vi "Report Get Gage Data.vi"(10 "Gage Data":string[][](array[string]), 11 "Array":dbl[][](array[numeric])) -> (1 "Array 2":i32[][](array[numeric]), 2 "Variant":variant, 3 "Array 3":string[][](array[string]))   [LabVIEW 2020]
uses:
  <vilib>/Analysis/baseanly.llb/Mean (DBL).vi
  <vilib>/Analysis/NI_AALBase.lvlib
panel:
  out "Variant 2":variant
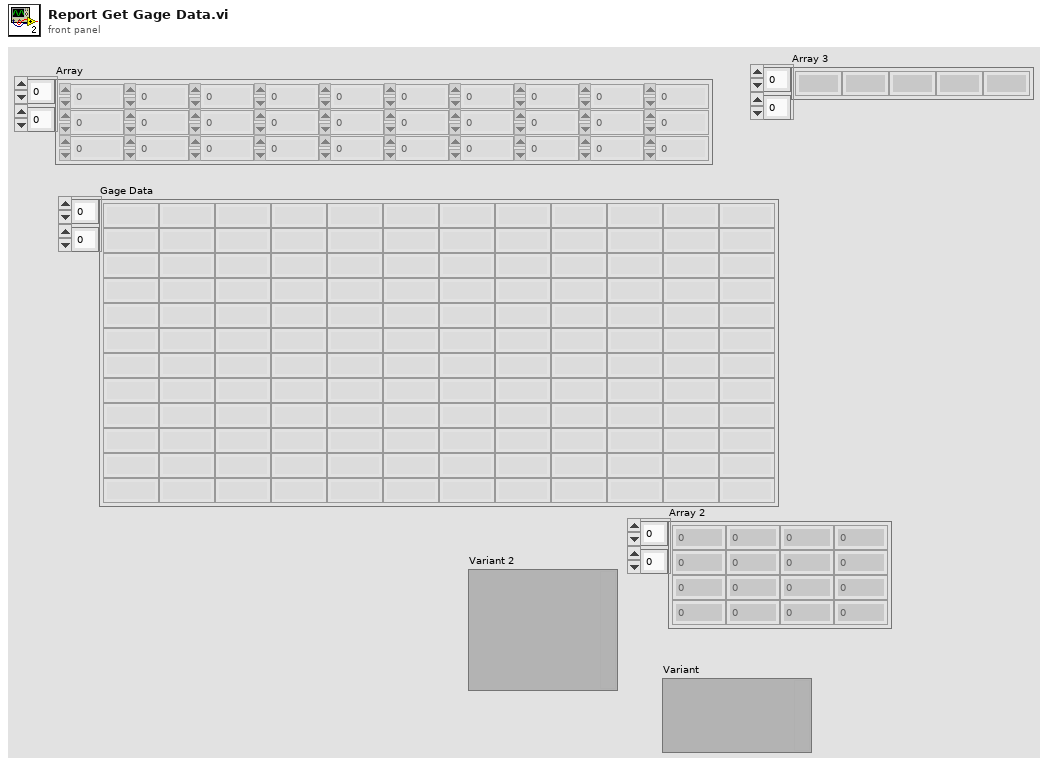
[diagram p1: front panel]
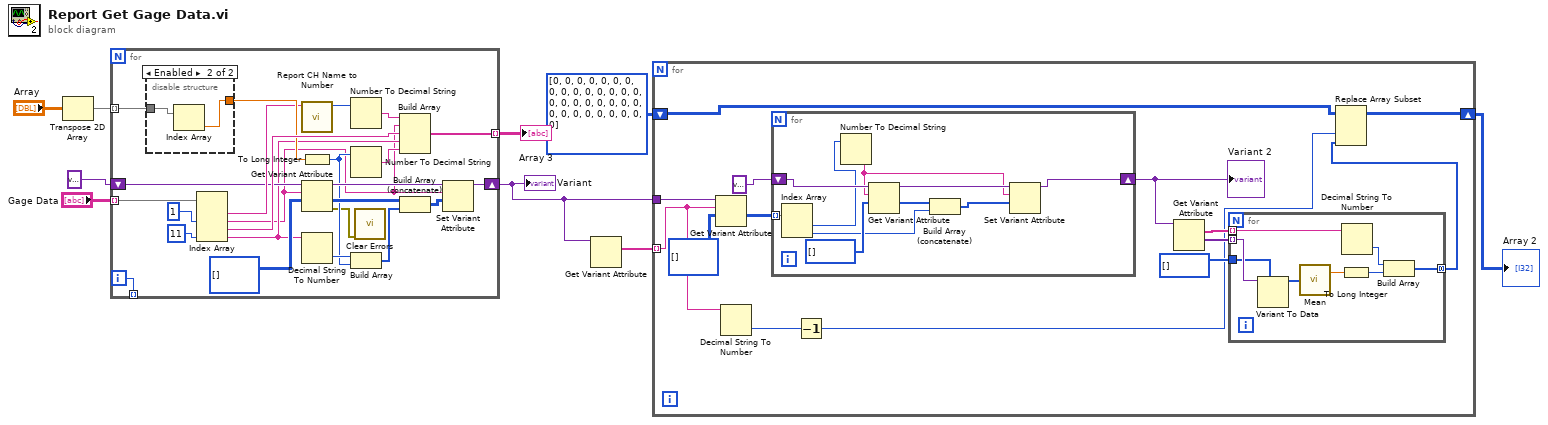
[diagram p0: block diagram]
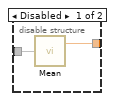
[diagram p2: hidden frame]
diagram:
  n1 = Transpose 2D Array(2D array="Array") -> (transposed array=w7:dbl[][])
  n2 = for {
    tunnel: "Gage Data" -> [w33] mode=indexing
    tunnel: [w28] -> w5 mode=indexing
    tunnel: w7 -> [w27] mode=indexing
    shift-right: [w17] -> w4
    shift-left: variant -> [w18]
    tunnel: [w11] -> _ mode=indexing
    i -> [w11]
    n3 = disable-structure shown="Enabled" {
      disable-tunnel: w27 -> [w35 w36]
      disable-tunnel: [w34 w37] -> w26
      frame Disabled {
        n4 = call-poly <vilib>:"Mean.vi"("X"=w35) -> ("mean"=w34:dbl)  [unwired: 1 out]
      }
      frame Enabled {
        n5 = Index Array(array=w36) -> (element=w37:dbl)  [unwired: 1 in]
      }
    }
    n6 = Index Array(array=w33, index #2=1 ("index"), index #4=11 ("index")) -> (element #1=w24:string, element #2=w12:string, element #3=w30:string, element #4=w16:string)  [unwired: 2 in]
    n7 = call "Report CH Name to Number.vi"("Ch Name"=w24) -> ("Ch number"=w23:i32)  [unwired: 10 in]
    n8 = To Long Integer(number=w26) -> (32bit integer=w14:i32)
    n9 = Get Variant Attribute(Variant=w18, name=w12, default value (empty Variant)=i32[][] [] ("index (row)")) -> (duplicate Variant=w20:variant, value=w21:i32[][], error out=w10:errorcluster)  [unwired: 1 in, 1 out]
    n10 = Decimal String To Number(string=w16) -> (number=w15:i32)  [unwired: 2 in, 1 out]
    n11 = Number To Decimal String(number=w23) -> (decimal integer string=w31:string)  [unwired: 1 in]
    n12 = Number To Decimal String(number=w14) -> (decimal integer string=w25:string)  [unwired: 1 in]
    n13 = Build Array(w15, w14) -> (w13:i32[])
    n14 = call <vilib>:"Clear Errors.vi"("error in (no error)"=w10) -> ()  [unwired: 5 in, 2 out]
    n15 = Build Array(w31, w12, w30, w16, w25) -> (w28:string[])
    n16 = Build Array (concatenate)(w21, w13) -> (w19:i32[][])
    n17 = Set Variant Attribute(Variant=w20, name=w12, value=w19) -> (Variant out=w17:variant)  [unwired: 1 in, 2 out]
  }
  "Variant" <- w4
  "Array 3" <- w5
  n18 = Get Variant Attribute(Variant=w4) -> (names=w3:string[])  [unwired: 3 in, 3 out]
  n19 = for {
    tunnel: w4 -> [w51]
    tunnel: w3 -> [w43] mode=indexing
    shift-right: [w39] -> w1
    shift-left: i32[][] [[0, 0, 0, 0], [0, 0, 0, 0], [0, 0, 0, 0], [0, 0, 0, 0], [0, 0, 0, 0], [0, 0, 0, 0], [0, 0, 0, 0], [0, 0, 0, 0]] ("index (row)") -> [w42]
    n20 = Get Variant Attribute(Variant=w51, name=w43, default value (empty Variant)=i32[][] [] ("index (row)")) -> (value=w49:i32[][])  [unwired: 1 in, 3 out]
    n21 = Decimal String To Number(string=w43) -> (number=w41:i32)  [unwired: 2 in, 1 out]
    n22 = for {
      tunnel: w49 -> [w67] mode=indexing
      shift-right: [w60] -> w47
      shift-left: variant -> [w69]
      n23 = Index Array(array=w67) -> (element #1=w66:i32, element #2=w63:i32)  [unwired: 2 in]
      n24 = Number To Decimal String(number=w66) -> (decimal integer string=w61:string)  [unwired: 1 in]
      n25 = Get Variant Attribute(Variant=w69, name=w61, default value (empty Variant)=i32[] [] ("index (row)")) -> (duplicate Variant=w68:variant, value=w64:i32[])  [unwired: 1 in, 2 out]
      n26 = Build Array (concatenate)(w64, w63) -> (w62:i32[])
      n27 = Set Variant Attribute(Variant=w68, name=w61, value=w62) -> (Variant out=w60:variant)  [unwired: 1 in, 2 out]
    }
    "Variant 2" <- w47
    n28 = Decrement(x=w41) -> (x-1=w38:i32)
    n29 = Get Variant Attribute(Variant=w47) -> (names=w44:string[], values=w46:variant[])  [unwired: 3 in, 2 out]
    n30 = for {
      tunnel: w46 -> [w59] mode=indexing
      tunnel: i32[] [] ("index (row)") -> [w58]
      tunnel: w44 -> [w56] mode=indexing
      tunnel: [w52] -> w40 mode=concatenating
      n31 = Variant To Data(type=w58, Variant=w59) -> (data=w57:i32[])  [unwired: 1 in, 1 out]
      n32 = call-poly <vilib>:"Mean.vi"("X"=w57) -> ("mean"=w55:dbl)  [unwired: 1 out]
      n33 = To Long Integer(number=w55) -> (32bit integer=w54:i32)
      n34 = Decimal String To Number(string=w56) -> (number=w53:i32)  [unwired: 2 in, 1 out]
      n35 = Build Array(w53, w54) -> (w52:i32[])
    }
    n36 = Replace Array Subset(array=w42, new element=w40, index (col)=w38) -> (w39:i32[][])  [unwired: 1 in]
  }
  "Array 2" <- w1
